vi "FindDataByCode.vi"(10 "Code":string, 11 "Database Path":path) -> (2 "all rows":string[](array[string]))   [LabVIEW 2014]
uses:
  <vilib>/Utility/file.llb/Read From Spreadsheet File (string).vi
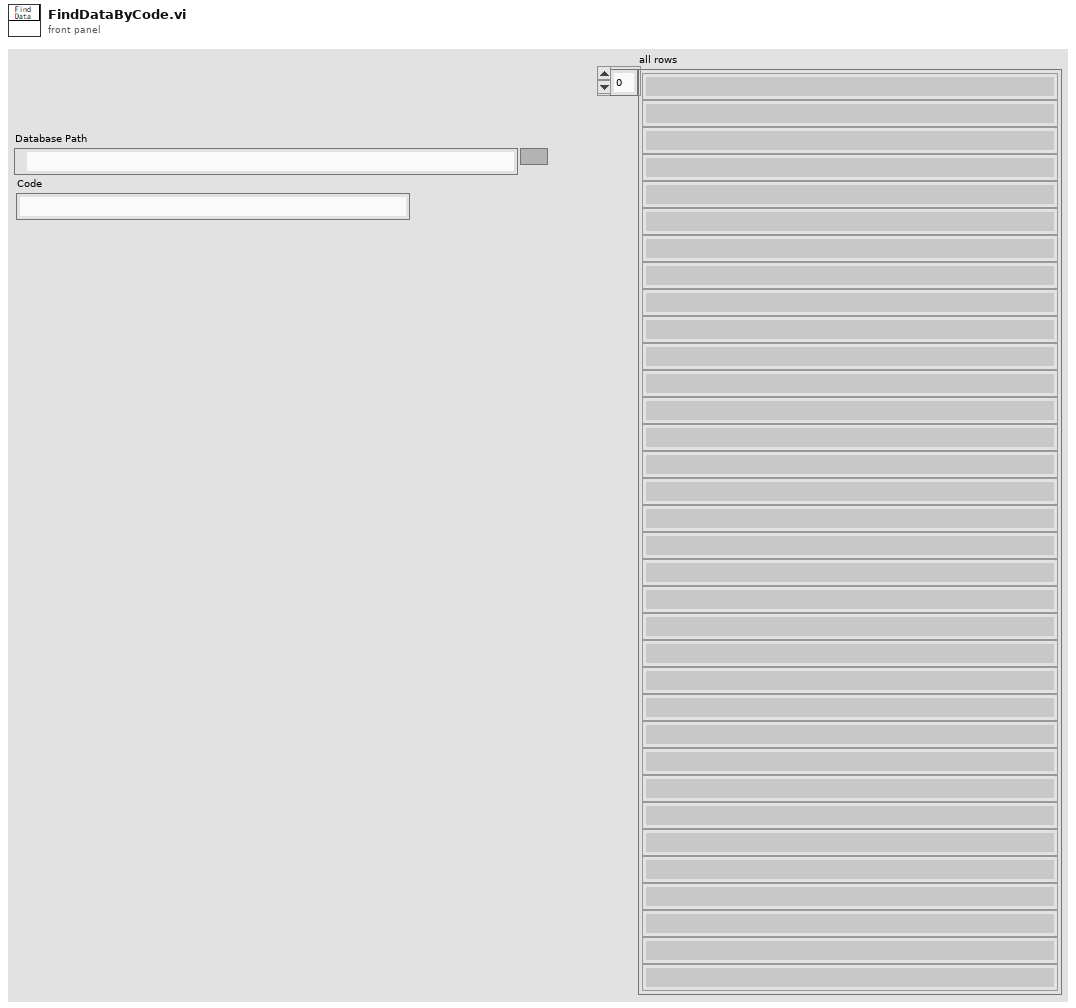
[diagram p1: front panel]
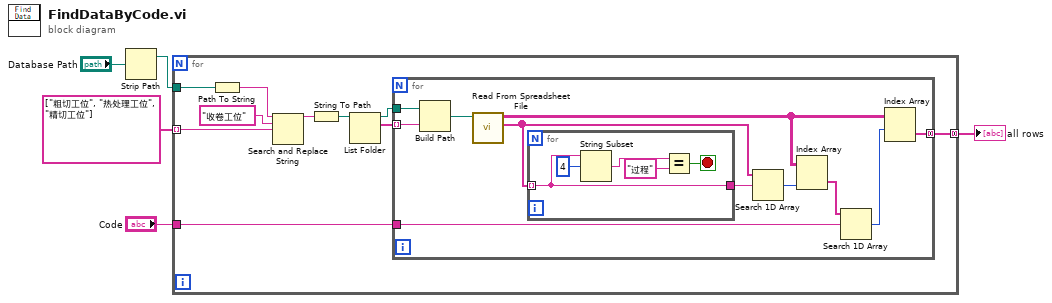
[diagram p0: block diagram]
diagram:
  n1 = Strip Path(path="Database Path") -> (stripped path=w4:path)  [unwired: 1 out]
  n2 = for {
    tunnel: w4 -> [w15]
    tunnel: string[] ["粗切工位", "热处理工位", "精切工位"] -> [w12] mode=indexing
    tunnel: "Code" -> [w7]
    tunnel: [w6] -> w1 mode=concatenating
    n3 = Path To String(path=w15) -> (string=w14:string)
    n4 = Search and Replace String(input string=w14, search string="收卷工位" ("搜索字符串"), replace string=w12) -> (result string=w11:string)  [unwired: 5 in, 3 out]
    n5 = String To Path(string=w11) -> (path=w10:path)
    n6 = List Folder(path=w10) -> (path out=w9:path, filenames=w8:string[])  [unwired: 3 in, 2 out]
    n7 = for {
      tunnel: w9 -> [w26]
      tunnel: w8 -> [w25] mode=indexing
      tunnel: w7 -> [w22]
      tunnel: [w18] -> w6 mode=concatenating
      n8 = Build Path(base path=w26, name or relative path=w25) -> (appended path=w19:path)
      n9 = call-poly <vilib>:"Read From Spreadsheet File.vi"("file path (dialog if empty)"=w19) -> ("first row"=w17:string[], "all rows"=w21:string[][])  [unwired: 6 in, 3 out]
      n10 = for {
        tunnel: w17 -> [w27] mode=indexing
        tunnel: [w27] -> w16
        stop <- w28 stop-if-true
        n11 = String Subset(string=w27, offset (0)=4 ("偏移量(0)")) -> (substring=w30:string)  [unwired: 1 in]
        n12 = Equal?(x=w30, y="过程" ("正则表达式")) -> (x = y?=w28:bool)
      }
      n13 = Search 1D Array(1D array=w17, element=w16) -> (index of element=w24:i32)  [unwired: 1 in]
      n14 = Index Array(array=w21, index (col)=w24) -> (element=w23:string[])  [unwired: 1 in]
      n15 = Search 1D Array(1D array=w23, element=w22) -> (index of element=w20:i32)  [unwired: 1 in]
      n16 = Index Array(array=w21, index (row)=w20) -> (element=w18:string[])  [unwired: 1 in]
    }
  }
  "all rows" <- w1
